vi "Parameter_read.vi"(7 "Para reference":T1, 10 "Array":u16[](array[numeric])) -> (3 "Para out":T1)   [LabVIEW 2017]
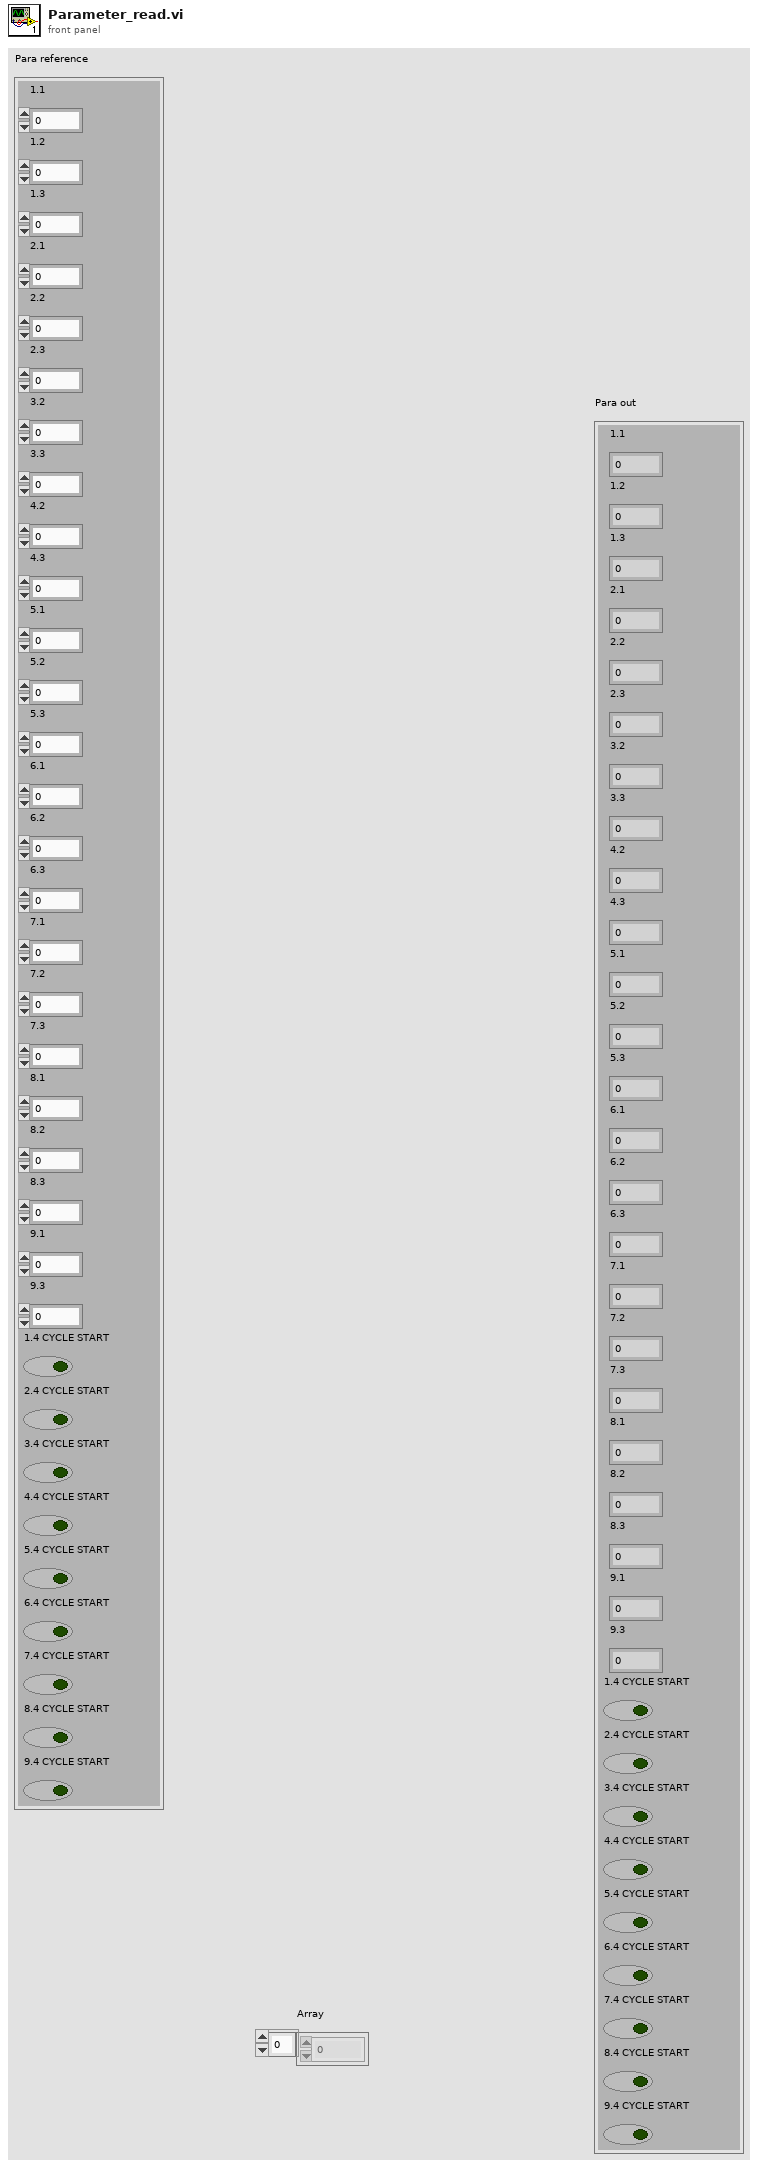
[diagram p1: front panel]
types:
  T1 = cluster{"1.1":dbl, "1.2":dbl, "1.3":dbl, "2.1":dbl, "2.2":dbl, "2.3":dbl, "3.2":dbl, "3.3":dbl, "4.2":dbl, "4.3":dbl, "5.1":dbl, "5.2":dbl, "5.3":dbl, "6.1":dbl, "6.2":dbl, "6.3":dbl, "7.1":dbl, "7.2":dbl, "7.3":dbl, "8.1":dbl, "8.2":dbl, "8.3":dbl, "9.1":dbl, "9.3":dbl, "1.4 CYCLE START":bool, "2.4 CYCLE START":bool, "3.4 CYCLE START":bool, "4.4 CYCLE START":bool, "5.4 CYCLE START":bool, "6.4 CYCLE START":bool, "7.4 CYCLE START":bool, "8.4 CYCLE START":bool, "9.4 CYCLE START":bool}
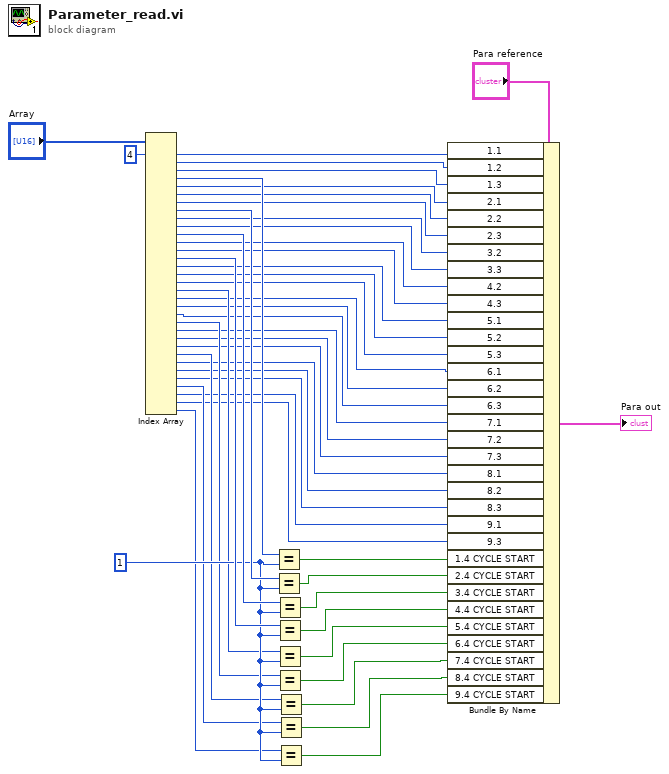
[diagram p0: block diagram]
diagram:
  w25 = 1 ("index")
  n1 = Index Array(array="Array", index #1=4 ("index")) -> (element #1=w45:u16, element #2=w46:u16, element #3=w47:u16, element #4=w41:u16, element #5=w40:u16, element #6=w39:u16, element #7=w38:u16, element #8=w35:u16, element #9=w33:u16, element #10=w32:u16, element #11=w31:u16, element #12=w30:u16, element #13=w29:u16, element #14=w27:u16, element #15=w19:u16, element #16=w18:u16, element #17=w17:u16, element #18=w16:u16, element #19=w15:u16, element #20=w14:u16, element #21=w13:u16, element #22=w12:u16, element #23=w11:u16, element #24=w10:u16, element #25=w9:u16, element #26=w8:u16, element #27=w7:u16, element #28=w6:u16, element #29=w5:u16, element #30=w4:u16, element #31=w3:u16, element #32=w2:u16, element #33=w1:u16)  [unwired: 32 in]
  n2 = Equal?(x=w41, y=w25) -> (x = y?=w36:bool)
  n3 = Equal?(x=w35, y=w25) -> (x = y?=w34:bool)
  n4 = Equal?(x=w31, y=w25) -> (x = y?=w28:bool)
  n5 = Equal?(x=w27, y=w25) -> (x = y?=w26:bool)
  n6 = Equal?(x=w16, y=w25) -> (x = y?=w24:bool)
  n7 = Equal?(x=w12, y=w25) -> (x = y?=w23:bool)
  n8 = Equal?(x=w8, y=w25) -> (x = y?=w22:bool)
  n9 = Equal?(x=w4, y=w25) -> (x = y?=w21:bool)
  n10 = Equal?(x=w1, y=w25) -> (x = y?=w20:bool)
  n11 = Bundle By Name(cluster="Para reference", "1.1"=w45, "1.2"=w46, "1.3"=w47, "2.1"=w40, "2.2"=w39, "2.3"=w38, "3.2"=w33, "3.3"=w32, "4.2"=w30, "4.3"=w29, "5.1"=w19, "5.2"=w18, "5.3"=w17, "6.1"=w15, "6.2"=w14, "6.3"=w13, "7.1"=w11, "7.2"=w10, "7.3"=w9, "8.1"=w7, "8.2"=w6, "8.3"=w5, "9.1"=w3, "9.3"=w2, "1.4 CYCLE START"=w36, "2.4 CYCLE START"=w34, "3.4 CYCLE START"=w28, "4.4 CYCLE START"=w26, "5.4 CYCLE START"=w24, "6.4 CYCLE START"=w23, "7.4 CYCLE START"=w22, "8.4 CYCLE START"=w21, "9.4 CYCLE START"=w20) -> (→"Para out":T1)
